vi "write and read paths.vi"(0 "Path":string, 11 "error in":errorcluster) -> (4 "Readed paths":string, 15 "error out":errorcluster)   [LabVIEW 2020, in "Custom Sort Function.lvlib"]
doc: "This VI is used to write and read paths from a text file and is used to give input to the other subVI"
uses:
  Custom Sort Function.lvlib
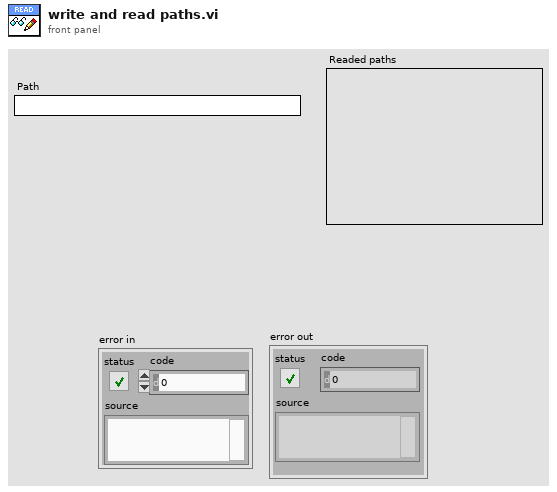
[diagram p1: front panel]
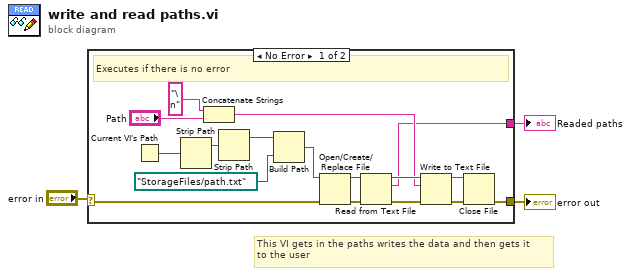
[diagram p0: block diagram]
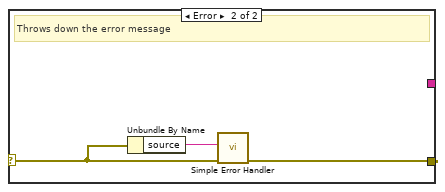
[diagram p2: hidden frame]
diagram:
  # "This VI gets in the paths writes the data and then gets it  \nto the user"
  n1 = case shown="No Error" "error in" {
    selector: "error in" -> [w7 w22]
    tunnel: [w12 w23] -> w3
    tunnel: [w4 _] -> w1
    frame No Error {
      # "Executes if there is no error"
      n2 = Current VI's Path() -> (path=w20:path)
      n3 = Strip Path(path=w20) -> (stripped path=w19:path)  [unwired: 1 out]
      n4 = Concatenate Strings("\n" ("string"), "Path") -> (w9:string)
      n5 = Strip Path(path=w19) -> (stripped path=w18:path)  [unwired: 1 out]
      n6 = Build Path(base path=w18, name or relative path=path "StorageFiles/path.txt") -> (appended path=w11:path)
      n7 = Open/Create/Replace File(file path (use dialog)=w11, error in=w7) -> (refnum out=w15:refnum<file>, error out=w16:errorcluster)  [unwired: 4 in, 1 out]
      n8 = Read from Text File(file (use dialog)=w15, error in=w16) -> (refnum out=w13:refnum<file>, text=w4:string, error out=w14:errorcluster)  [unwired: 2 in, 1 out]
      n9 = Write to Text File(file (use dialog)=w13, text=w9, error in=w14) -> (refnum out=w6:refnum<file>, error out=w5:errorcluster)  [unwired: 1 in, 1 out]
      n10 = Close File(refnum=w6, error in=w5) -> (error out=w12:errorcluster)  [unwired: 1 out]
    }
    frame Error {
      # "Throws down the error message"
      n11 = Unbundle By Name(w22) -> ("source"=w21:string)
      n12 = call <vilib>:"Simple Error Handler.vi"("error source (\" \")"=w21, "error in (no error)"=w22) -> ("error out"=w23:errorcluster)  [unwired: 3 in, 4 out]
    }
  }
  "error out" <- w3
  "Readed paths" <- w1
